vi "c_ctre_phoenix6_get_signal.vi"(0 "Numeric 2":u32, 1 "Cluster":cluster{"deviceHash":u32, "spn":u32}, 2 "String 2":string, 3 "Numeric 3":u8, 4 "Numeric 4":dbl) -> (20 "Numeric":i32, 21 "Cluster 2":T1, 22 "String":string)   [LabVIEW 2023]
uses:
  <vilib>/Rock Robotics/WPI/ThirdParty/Phoenix-LabVIEW/Controls/DriverLib.ctl
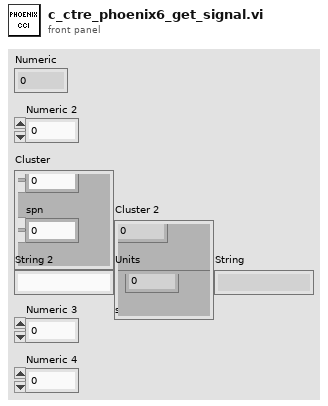
[diagram p1: front panel]
types:
  T1 = cluster{"OutValue":dbl, "Units":cluster{"Numeric":u8, "Numeric 2":u8, "Numeric 3":u8, "Numeric 4":u8, "Numeric 5":u8, "Numeric 6":u8, "Numeric 7":u8, "Numeric 8":u8, "Numeric 9":u8, "Numeric 10":u8}, "swTimestampSeconds":dbl, "hwTimestampSeconds":dbl, "ecuTimestampSeconds":dbl, "error":i32}
  T2 = cluster{"OutValue":dbl, "Units":cluster{u8, u8, u8, u8, u8, u8, u8, u8, u8, u8}, "swTimestampSeconds":dbl, "hwTimestampSeconds":dbl, "ecuTimestampSeconds":dbl, "error":i32}
  T3 = typedef "DriverLib.ctl" = path
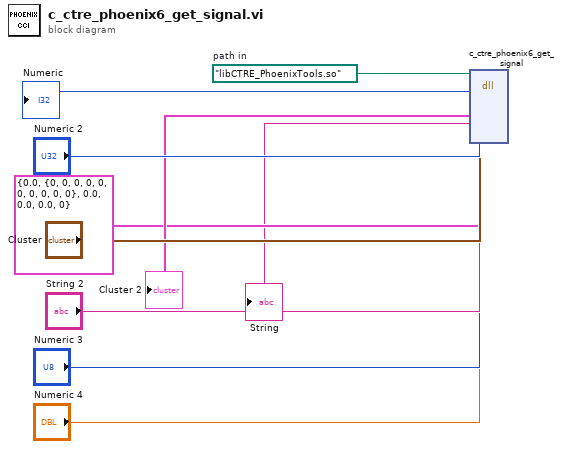
[diagram p0: block diagram]
diagram:
  w10 = T3 path "libCTRE_PhoenixTools.so"  # path in
  n1 = dll-call lib="?" fn="c_ctre_phoenix6_get_signal"(path in=w10, "Numeric 2", "Cluster", "Cluster 2"=T2 {"OutValue"=0.0, "Units"={0, 0, 0, 0, 0, 0, 0, 0, 0, 0}, "swTimestampSeconds"=0.0, "hwTimestampSeconds"=0.0, "ecuTimestampSeconds"=0.0, "error"=0}, "String 2", "Numeric 3", "Numeric 4") -> (→"Numeric":i32, "Cluster 2"=→"Cluster 2":T2, →"String":string)  [unwired: 6 in, 2 out]
